vi "Reconstruct_from_patches_2d.vi"(8 "error in":errorcluster caption="entrée d'erreur", 10 "patches":cluster{"Array":i32[][]}[](array[cluster])) -> (0 "error out":errorcluster caption="sortie d'erreur", 3 "Data":T1)   [LabVIEW 2020]
uses:
  Reconstruct_from_patches_2d.lvclass
panel:
  in  "image_size":cluster{"image_height":i32, "image_width":i32}
  out "Reconstruct_from_patches_2d.lvclass":refnum<class "Reconstruct_from_patches_2d.lvclass">
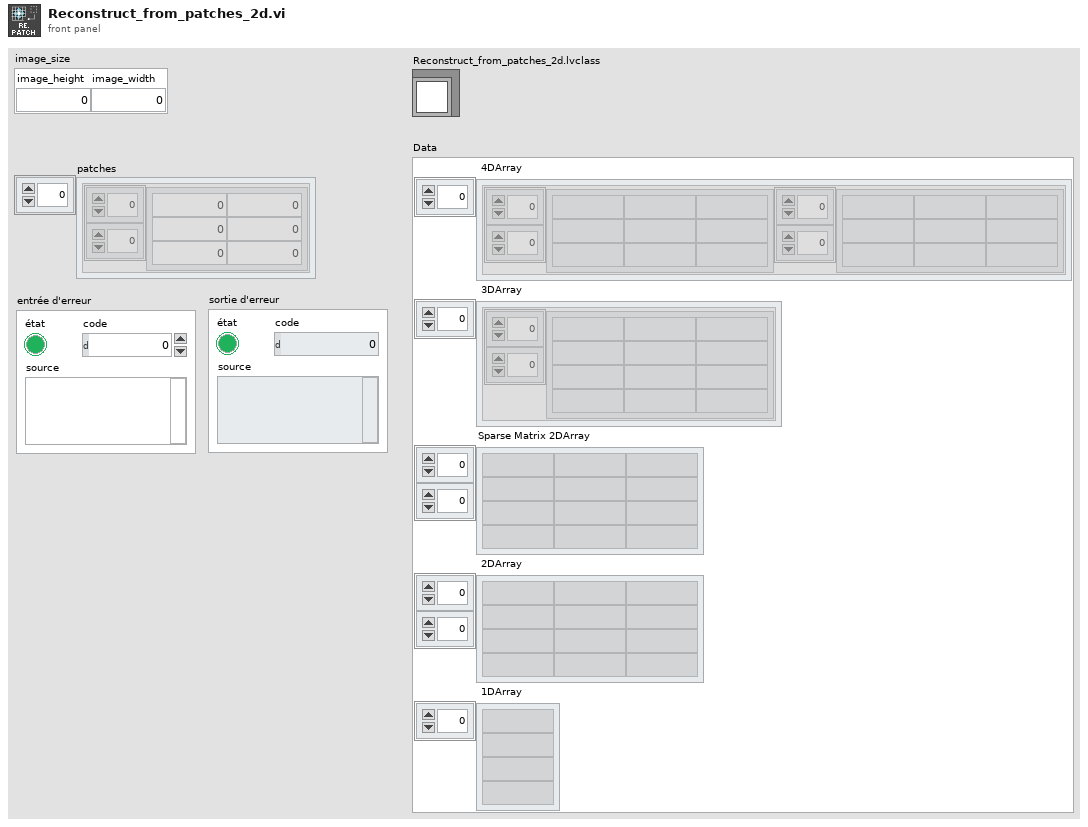
[diagram p1: front panel]
types:
  T1 = cluster{" 4DArray":cluster{"1":string[][], "2":string[][]}[], " 3DArray":cluster{"Tableau":string[][]}[], "Sparse Matrix 2DArray":string[][], " 2DArray":string[][], " 1DArray":string[]}
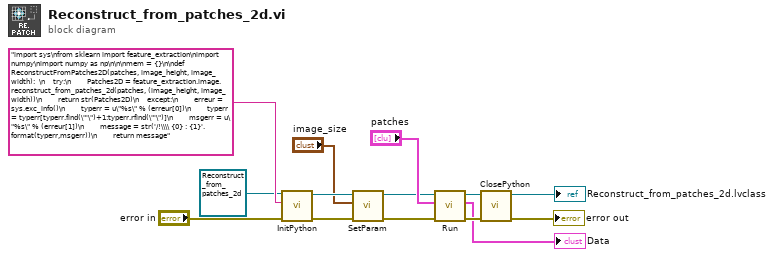
[diagram p0: block diagram]
diagram:
  n1 = call-dynamic "InitPython.vi"("error in (no error)"="error in", "Python Instruction"="import sys\nfrom sklearn import feature_extraction\nimport numpy\nimport numpy as np\n\n\nmem = {}\n\ndef ReconstructFromPatches2D(patches, image_height, image_width):  \n    try:\n        Patches2D = feature_extraction.image.reconstruct_from_patches_2d(patches, (image_height, image_width))\n        return str(Patches2D)\n    except:\n        erreur = sys.exc_info()\n        typerr = u\"%s\" % (erreur[0])\n        typerr = typerr[typerr.find(\"'\")+1:typerr.rfind(\"'\")]\n        msgerr = u\"%s\" % (erreur[1])\n        message = str('/!\\\\ {0} : {1}'. format(typerr,msgerr))\n        return message", "Scikit-learn en entrée"=refnum<class "Reconstruct_from_patches_2d.lvclass"> refnum ("Reconstruct_from_patches_2d.lvclass")) -> ("error out"=w4:errorcluster, "Scikit-learn en sortie"=w5:refnum<class "Reconstruct_from_patches_2d.lvclass">)  [unwired: 7 in]
  n2 = call-dynamic "SetParam.vi"("error in (no error)"=w4, "image_size"="image_size", "Reconstruct_from_patches_2d in"=w5) -> ("error out"=w2:errorcluster, "Reconstruct_from_patches_2d out"=w3:refnum<class "Reconstruct_from_patches_2d.lvclass">)  [unwired: 7 in]
  n3 = call-dynamic "Run.vi"("error in (no error)"=w2, "patches"="patches", "Reconstruct_from_patches_2d.lvclass"=w3) -> ("error out"=w11:errorcluster, "Data"=→"Data":T1, "Reconstruct_from_patches_2d.lvclass"=w10:refnum<class "Reconstruct_from_patches_2d.lvclass">)  [unwired: 6 in]
  n4 = call-dynamic "ClosePython.vi"("error in (no error)"=w11, "Scikit-learn en entrée"=w10) -> ("error out"=→"error out":errorcluster, "Scikit-learn en sortie"=→"Reconstruct_from_patches_2d.lvclass":refnum<class "Reconstruct_from_patches_2d.lvclass">)  [unwired: 8 in]
